vi "Write hostLoopPeriodAllowedJitter_percent.vi"(8 "error in (no error)":errorcluster, 10 "hostLoopPeriodAllowedJitter_percent":dbl=10.0, 11 "LoopConfig in":refnum<class "LoopConfig.lvclass">) -> (0 "error out":errorcluster, 3 "LoopConfig out":refnum<class "LoopConfig.lvclass">)   [LabVIEW 2013, in "ComponentData.lvlib" / "LoopConfig.lvclass"]
uses:
  <userlib>/Common/Component/Application/RT/ComponentData/ConfigurationHandler/LoopConfig/LoopConfig.lvclass
  <userlib>/Common/Component/Application/RT/ComponentData/ConfigurationHandler/LoopConfig/LoopConfig.lvclass/LoopConfig.ctl
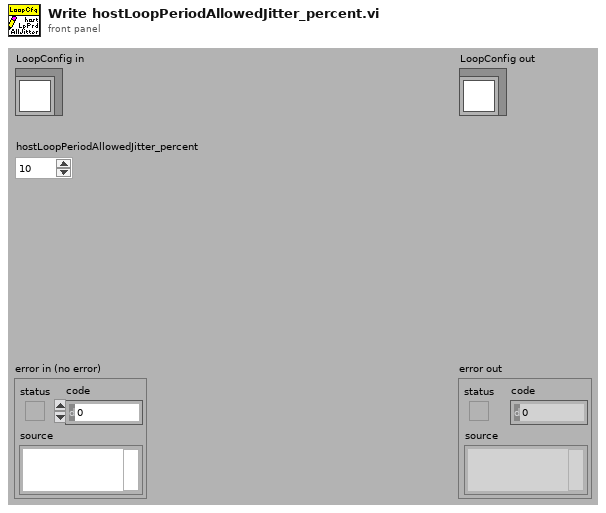
[diagram p1: front panel]
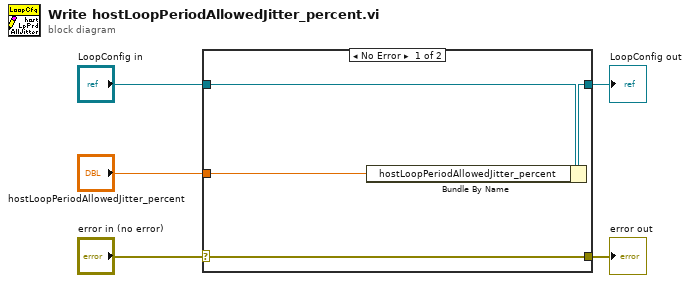
[diagram p0: block diagram]
diagram:
  n1 = case shown="No Error" "error in (no error)" {
    selector: "error in (no error)" -> [w9 w10]
    tunnel: [w9 w10] -> w4
    tunnel: [w7 w11] -> w2
    tunnel: "LoopConfig in" -> [w8 w11]
    tunnel: "hostLoopPeriodAllowedJitter_percent" -> [w6 _]
    frame No Error {
      n2 = Bundle By Name(cluster=w8, "hostLoopPeriodAllowedJitter_percent"=w6) -> (w7:refnum<class "LoopConfig.lvclass">)
    }
    frame Error {
    }
  }
  "error out" <- w4
  "LoopConfig out" <- w2
